vi "Test Convert.vi"(8 "error in (no error)":errorcluster, 11 "Temperature Converter Test In":refnum<class "Temperature Converter Test.lvclass">) -> (0 "error out":errorcluster, 3 "Temperature Converter Test Out":refnum<class "Temperature Converter Test.lvclass">)   [LabVIEW 2020, in "Temperature Converter Test.lvclass"]
uses:
  Temperature Converter Test.lvclass
  C:/Program Files (x86)/National Instruments/LabVIEW 2020/vi.lib/Astemes/LUnit/Test Case.lvclass
  Temperature Converter Test.lvclass/Temperature Converter Test.ctl
  <vilib>/Astemes/LUnit/Test Case.lvclass/Test Case.ctl
  d3deb2a1-d8de-4edf-9525-d8a4abe28bdc.vi
  <vilib>/Astemes/LUnit/Append Pass Result.vi
  <vilib>/Astemes/LUnit/Append Fail Result.vi
  <vilib>/Astemes/LUnit/Describe Comparison.vi
  <vilib>/Astemes/LUnit/Compare Variants.vi
  <vilib>/Astemes/LUnit/Run In UI.vi
  <vilib>/Utility/error.llb/Clear Errors.vi
  <vilib>/Astemes/LUnit/Describe Variant.vi
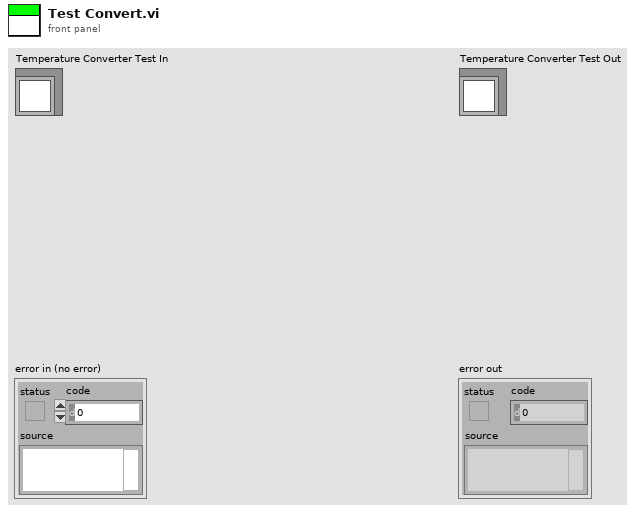
[diagram p1: front panel]
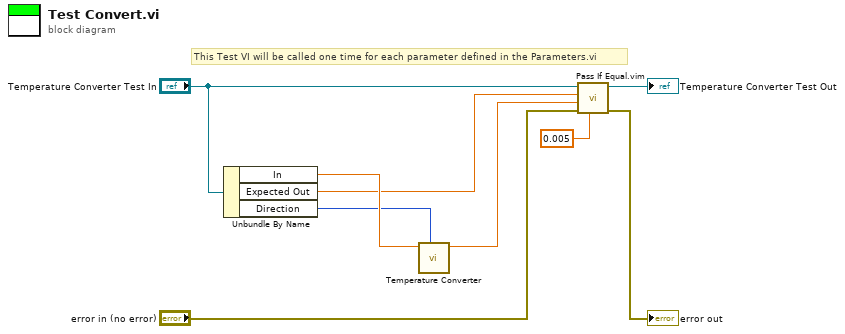
[diagram p0: block diagram]
diagram:
  # "This Test VI will be called one time for each parameter defined in the Parameters.vi"
  n1 = Unbundle By Name("Temperature Converter Test In") -> ("In"=w9:dbl, "Expected Out"=w2:dbl, "Direction"=w8:enum16{"F to C", "C to F"})
  n2 = call "Temperature Converter.vi"("Direction"=w8, "In"=w9) -> ("Out"=w3:dbl)  [unwired: 9 in]
  n3 = call "Pass If Equal.vim"("Delta"=0.005 ("Out"), "error in (no error)"="error in (no error)", "Actual"=w3, "Expected"=w2, "LUnit Test Case In"="Temperature Converter Test In") -> ("error out"=→"error out":errorcluster, "LUnit Test Case Out"=→"Temperature Converter Test Out":refnum<class "Temperature Converter Test.lvclass">)  [unwired: 5 in]
